vi "test philosopher.vi"() -> ()   [LabVIEW 2023, in "Philosopher.lvlib"]
uses:
  Philosopher.lvlib
  Philosopher/Philosopher.lvclass
  C:/Program Files (x86)/National Instruments/LabVIEW 2023/vi.lib/ActorFramework/Actor/Actor.lvclass
  <vilib>/Utility/miscctls.llb/LVRectTypeDef.ctl
  Philosopher Messages/Assigned seat/Assigned seat Msg.lvclass/Assigned seat Msg.ctl
  <vilib>/ActorFramework/Message Enqueuer/Message Enqueuer.lvclass/Message Enqueuer.ctl
  <vilib>/ActorFramework/Message Enqueuer/Enqueue.vi
  Philosopher Messages/Assigned seat/Assigned seat Msg.lvclass
  C:/Program Files (x86)/National Instruments/LabVIEW 2023/vi.lib/ActorFramework/Message/Message.lvclass
  Philosopher Messages/Timeout Hungry/Timeout Eating Msg.lvclass
  Philosopher Messages/Go to eating/Eat.lvclass
  <vilib>/ActorFramework/Stop Msg/Stop Msg.lvclass
  <vilib>/ActorFramework/Message Priority Queue/Priority Enqueue.vi
  <vilib>/ActorFramework/Actor/Actor.lvclass
panel:
  in  "stop":bool
  in  "Eat":bool
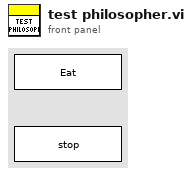
[diagram p1: front panel]
types:
  T1 = typedef "LVRectTypeDef.ctl" = cluster{"Left":i16, "Top":i16, "Right":i16, "Bottom":i16}
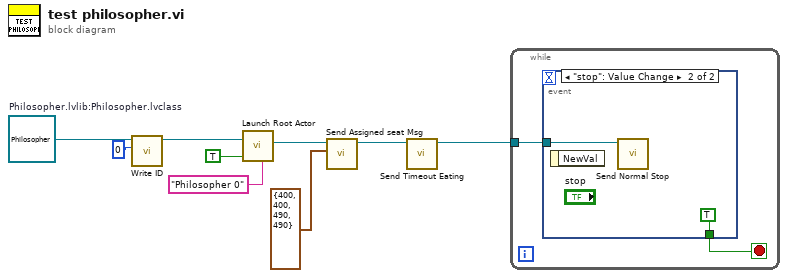
[diagram p0: block diagram]
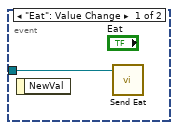
[diagram p2: hidden frame]
diagram:
  w7 = refnum<class "Philosopher.lvclass"> refnum  # Philosopher.lvlib:Philosopher.lvclass
  n1 = call-dynamic "Write ID.vi"("ID"=0, "Philosopher in"=w7) -> ("Philosopher out"=w6:refnum<class "Philosopher.lvclass">)  [unwired: 8 in, 1 out]
  n2 = call <vilib>:"Launch Root Actor.vi"("Debug Alias"="Philosopher 0", "Open Actor Core front panel? (F)"=TRUE, "Actor"=w6) -> ("Actor's Enqueuer"=w4:refnum<class "Message Enqueuer.lvclass">)  [unwired: 7 in, 1 out]
  n3 = call "Send Assigned seat Msg.vi"("Front Panel Window:Panel Bounds"=T1 {"Left"=400, "Top"=400, "Right"=490, "Bottom"=490}, "Message Enqueuer"=w4) -> ("Message Enqueuer"=w2:refnum<class "Message Enqueuer.lvclass">)  [unwired: 8 in, 1 out]
  n4 = call "Send Timeout Eating.vi"("Message Enqueuer"=w2) -> ("Message Enqueuer"=w1:refnum<class "Message Enqueuer.lvclass">)  [unwired: 9 in, 1 out]
  n5 = while {
    tunnel: w1 -> [w11]
    stop <- w10 stop-if-true
    n6 = event shown="[1] \"stop\": Value Change" {
      selector: _ -> [_ _]
      dyn-events: _ -> [_ _]
      timeout: _ -> [_ _]
      tunnel: w11 -> [w12 w14]
      tunnel: [_ TRUE] -> w10
      event "Eat": Value Change {
        n7 = event-data() -> ()  [unwired: 1 in, 1 out]
        n8 = call "Send Eat.vi"("Message Enqueuer"=w12) -> ()  [unwired: 9 in, 2 out]
      }
      event "stop": Value Change {
        n9 = event-data() -> ()  [unwired: 1 in, 1 out]
        n10 = call <vilib>:"Send Normal Stop.vi"("Message Enqueuer"=w14) -> ()  [unwired: 10 in, 1 out]
      }
    }
  }
